vi "InstrumentControlExercises_MichaelVasmerDavidWise.vi"() -> ()   [LabVIEW 2012]
doc: "This example shows how to configure a measurement and take a reading."
uses:
  Program Files (x86)/National Instruments/LabVIEW 2013/instr.lib/Keithley 24XX/Keithley 24XX.lvlib
  <vilib>/express/express arith-compare/Formula/XNode/ExpressFormulaBlockNode.xnode
  Control2_MichaelVasmerDavidWise.ctl
  He3_Tlogger_Global 1.vi
  Control3_MichaelVasmerDavidWise.ctl
  Program Files (x86)/National Instruments/LabVIEW 2013/instr.lib/Stanford Research 830/Stanford Research 830.lvlib
  Program Files (x86)/National Instruments/LabVIEW 2013/instr.lib/Keithley 24XX/Public/Data/Read (Single Point).vi
  Program Files (x86)/National Instruments/LabVIEW 2013/instr.lib/Stanford Research 830/Public/Data/Read (All Parameters).vi
  <vilib>/Utility/file.llb/Write To Spreadsheet File (string).vi
  <vilib>/Utility/file.llb/Write To Spreadsheet File (DBL).vi
panel:
  out "Step constant":dbl
  out "Forwards":bool
  out "Array":dbl[](array[numeric])=[0.002, 0.004, 0.006, 0.008, 0.01, 0.012, 0.014, 0.016, 0.018000000000000002, 0.02, 0.022, 0.024, 0.026000000000000002, 0.028]
  out "error out":errorcluster
  out "VISA resource name out":refnum<visa-resource-name>="Keithley"
  in  "Compliance  Level (0.1)":dbl=4.0
  out "Keithley Input Current (A)":dbl=0.4222222222222222
  out "T 2":dbl=293.425
  out "T 1":dbl=293.425
  out "V_output_Y_channel":dbl
  out "V_output_X_channel":dbl=0.0153199
  in  "R Series Value":dbl=100000.0
  in  "True  = R(B)\nFalse = R(T)":bool
  in  "Lock In On (default false)":bool
  out "Outer State Machine":T1=enum."Idle"
  out "Inner State Machine":T2=enum."Idle"
  out "I_AC Amplitude (A)":dbl=1e-05
  in  "Keithley on (default false)":bool
  out "Magnetic Field (T)":dbl
  in  "Internal Reference Frequency (1000 Hz)":dbl=1573.0
  in  "Sine Output Amplitude (1 V)":dbl=1.0
  in  "Sensitivity (26: 1 V/uA)":i8(ring)=26 items=["Auto Gain"=-1, "2 nV/fA"=0, "5 nV/fA"=1, "10 nV/fA"=2, "20 nV/fA"=3, "50 nV/fA"=4, "100 nV/fA"=5, "200 nV/fA"=6, "500 nV/fA"=7, "1 uV/pA"=8, "2 uV/pA"=9, "5 uV/pA"=10, "10 uV/pA"=11, "20 uV/pA"=12, "50 uV/pA"=13, "100 uV/pA"=14, "200 uV/pA"=15, "500 uV/pA"=16, "1 mV/nA"=17, "2 mV/nA"=18, "5 mV/nA"=19, "10 mV/nA"=20, "20 mV/nA"=21, "50 mV/nA"=22, "100 mV/nA"=23, "200 mV/nA"=24, "500 mV/mA"=25, "1 V/uA"=26]
  in  "Dynamic Reserve (2: Low Noise)":i8(ring)=2 items=["High Reserve"=0, "Normal"=1, "Low Noise"=2, "Auto Reserve"=-1]
  in  "Reference Source (1: Internal)":u16(ring)=1 items=["External", "Internal"]
  in  "Input Coupling (0: AC)":u16(ring) items=["AC", "DC"]
  in  "Input Connection (0: Single-Ended Voltage)":u16(ring) items=["Single-Ended Voltage", "Differential Voltage", "1 MOhm Current Gain", "100 MOhm Current Gain"]
  in  "VISA resource name Lock-In":refnum<visa-resource-name>="LockIn"
  out "Temperature (K)":dbl=293.453
  in  "Shutdown":bool
  out "Resistance":sgl=13619.99
  out "Current":sgl=0.00029368006
  out "Voltage":sgl=3.9999197
  in  "Enable Resistance Auto Range (T:Enable)":bool=TRUE
  in  "Enable Current Auto Range (T:Enable)":bool=TRUE
  in  "Enable Voltage Auto Range (T:Enable)":bool=TRUE
  in  "Resistance Manual Range (1.0)":dbl=1.0
  in  "Current Manual Range (1.0)":dbl=1.0
  in  "Voltage Manual Range (1.0)":dbl=1.0
  in  "Serial Configuration":T3={"Baud Rate"=9600, "Parity"=0, "Data Bits"=8, "Stop Bits"=10, "Flow Control"=0} {"Flow Control" items=["None", "XON/XOFF", "RTS/CTS", "XON/XOFF & RTS/CTS", "DTR/DSR", "XON/XOFF & DTR/DSR"]; "Stop Bits" items=["1.0"=10, "1.5"=15, "2.0"=20]; "Data Bits" items=["7"=7, "8"=8]; "Parity" items=["None", "Odd", "Even", "Mark", "Space"]; "Baud Rate" items=["300"=300, "600"=600, "1200"=1200, "2400"=2400, "4800"=4800, "9600"=9600, "19200"=19200]}
  in  "VISA resource name Kiethley":refnum<visa-resource-name>="Keithley"
  in  "Tab Control":enum32{" R(B)", "R(T)"}(tab)=enum."R(T)"
  in  "Time Delay":dbl=2.0
  out "Field too high error":string
  in  "Sweep R(B)":bool
  in  "B Max\n|B|<0.0716":dbl=0.03 step=0.01
  in  "File String Template":string="C:\\Users\\Josephson Lab User\\Documents\\CDT_2016\\MichaelDavid\\data\\test_RB"
  out "R vs B":cluster{dbl[], dbl[]}(graph)={[0.002, 0.004, 0.006, 0.008, 0.01, 0.012, 0.014, 0.016, 0.018000000000000002, 0.02, 0.022, 0.024, 0.026000000000000002, 0.028, 0.029999999999999995], [1531.9899999999998, 1531.9899999999998, 1531.9899999999998, 1531.9899999999998, 1531.9899999999998, 1531.9899999999998, 1531.9899999999998, 1531.9899999999998, 1531.9899999999998, 1531.9899999999998, 1531.9899999999998, 1531.9899999999998, 1531.9899999999998, 1531.9899999999998, 1531.9899999999998]}
  in  "Steps":dbl=15.0
  in  "Sweep R(T)":bool
  in  "Stop Sweep R(T)":bool
  in  "Force Measurement":bool
  in  "File String Template 2":string="C:\\Users\\Josephson Lab User\\Documents\\CDT_2016\\MichaelDavid\\data\\test_RT"
  out "R vs Temp":cluster{dbl[], dbl[]}(graph)={[293.427, 293.452, 293.456, 293.434, 293.429, 293.426, 293.438, 293.446, 293.454, 293.431, 293.461, 293.42, 293.423, 293.447, 293.466, 293.452, 293.463, 293.456, 293.44, 293.45, 293.434, 293.442, 293.425], [1531.9899999999998, 1531.9899999999998, 1531.9899999999998, 1531.9899999999998, 1531.9899999999998, 1531.9899999999998, 1531.9899999999998, 1531.9899999999998, 1531.9899999999998, 1531.9899999999998, 1531.9899999999998, 1531.9899999999998, 1531.9899999999998, 1531.9899999999998, 1531.9899999999998, 1531.9899999999998, 1531.9899999999998, 1531.9899999999998, 1531.9899999999998, 1531.9899999999998, 1531.9899999999998, 1531.9899999999998, 1531.9899999999998]}
  # "Keithley Settings"
  # "Voltage Range Settings"
  # "Current Range Settings"
  # "Resistance Range Settings"
  # "SR830 Lock In Settings"
  # "Keithley Output"
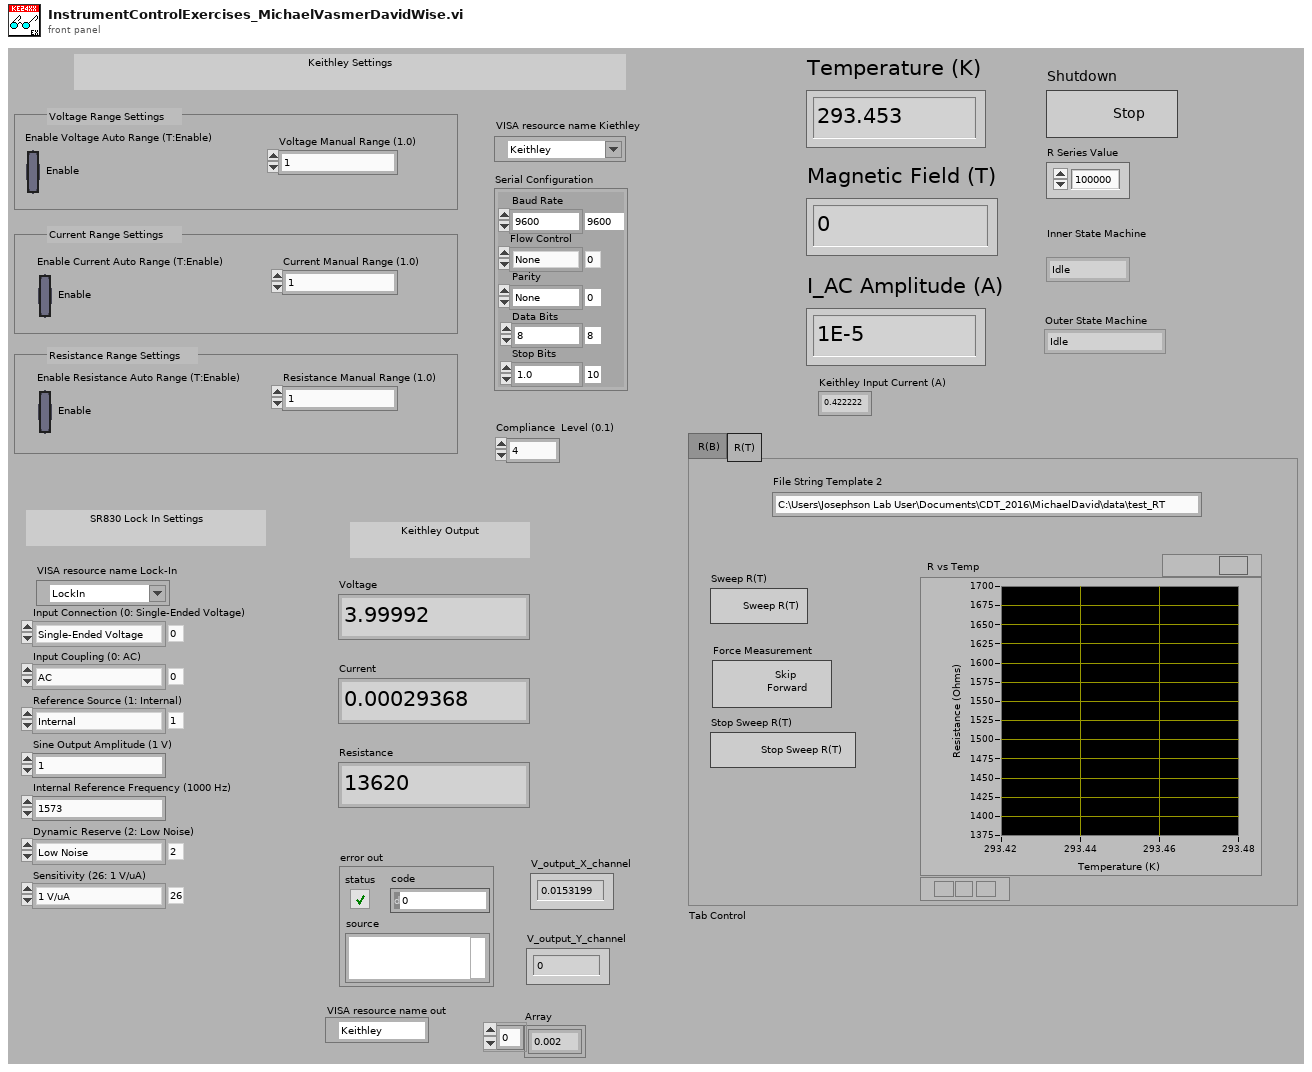
[diagram p1: front panel]
types:
  T1 = typedef "Control2_MichaelVasmerDavidWise.ctl" = enum16{"Open File 2", "Write File", "Open File", "Shutdown All", "Shutdown Lock in", "Read R(T)", "Init Lock In", "Increment", "Shutdown Keithley", "Idle", "Exit", "Read R(B)", "Set B", "Init Keithley"}
  T2 = typedef "Control3_MichaelVasmerDavidWise.ctl" = enum16{"Write File", "Read T 2", "Idle", "Read Lockin", "Read T"}
  T3 = cluster{"Baud Rate":u32, "Parity":u16, "Data Bits":u16, "Stop Bits":u16, "Flow Control":u16}
  T4 = cluster{"X-Value":dbl, "Y-Value":dbl, "R-Value":dbl, "Theta-Value":dbl, "Aux In 1 Value":dbl, "Aux In 2 Value":dbl, "Aux In 3 Value":dbl, "Aux In 4 Value":dbl, "Reference Frequency":dbl, "Channel 1 Display":dbl, "Channel 2 Display":dbl}
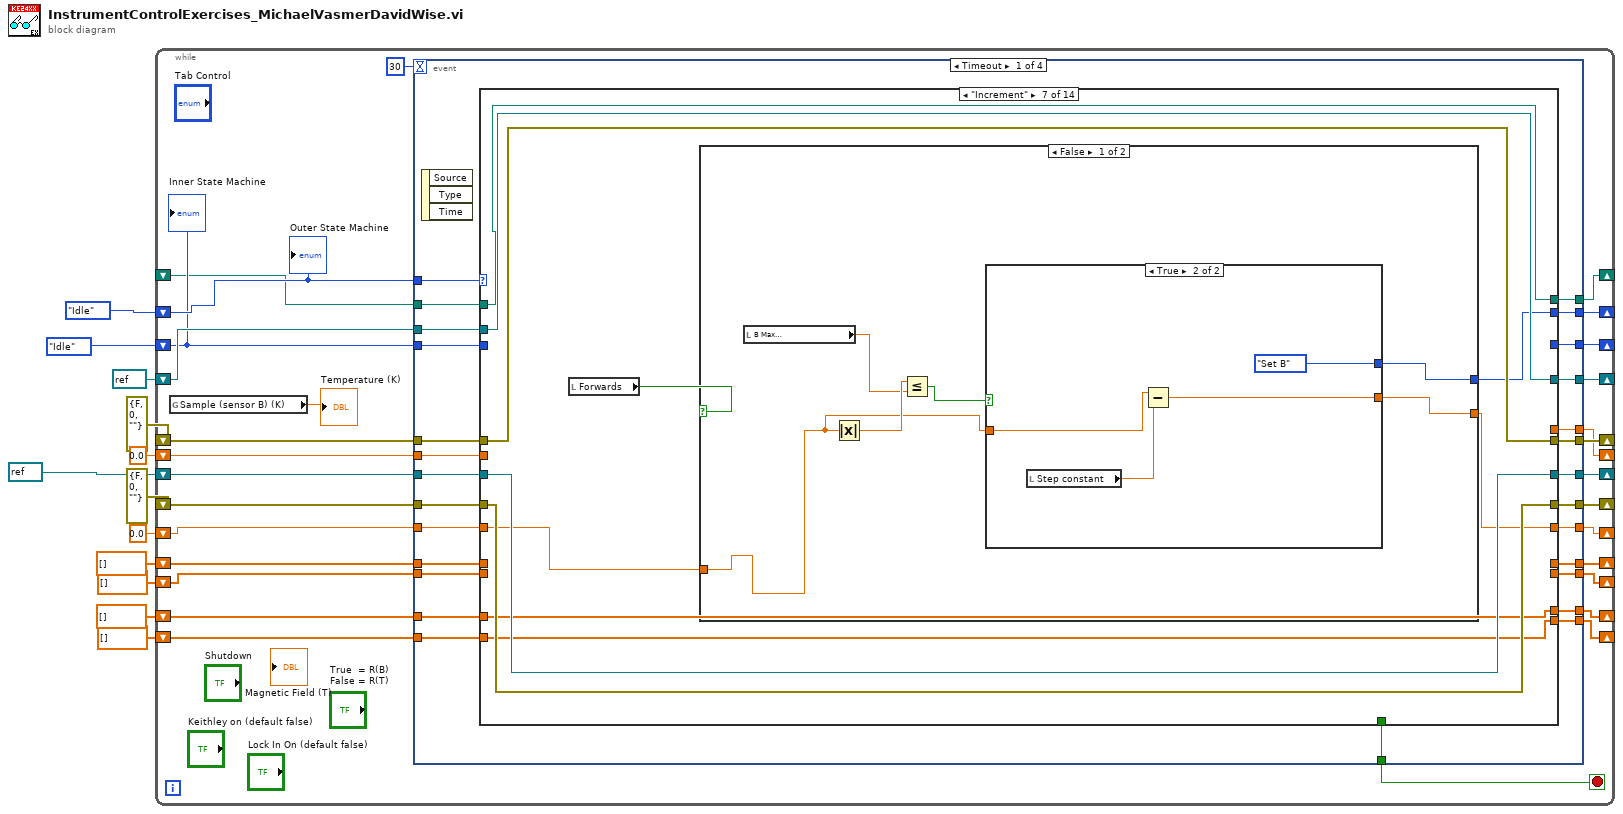
[diagram p0: block diagram]
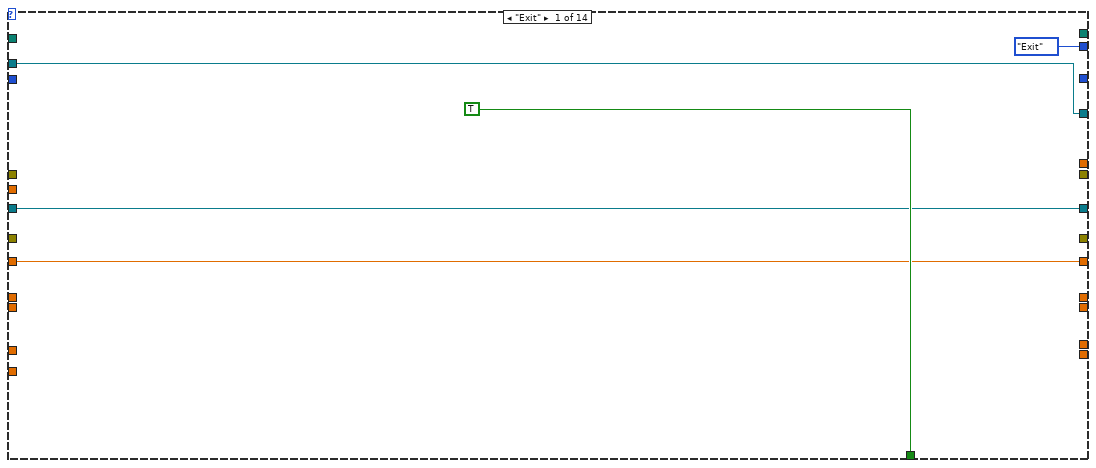
[diagram p2: hidden frame]
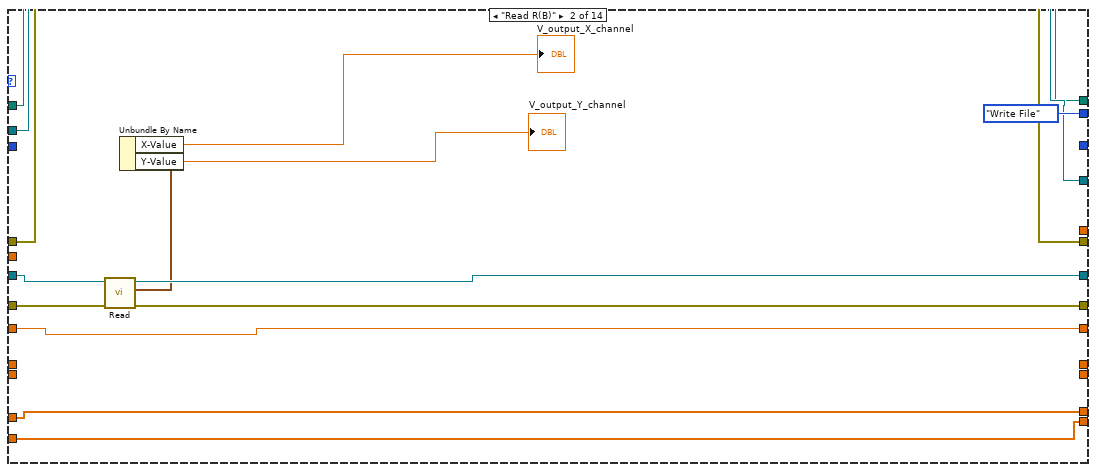
[diagram p3: hidden frame]
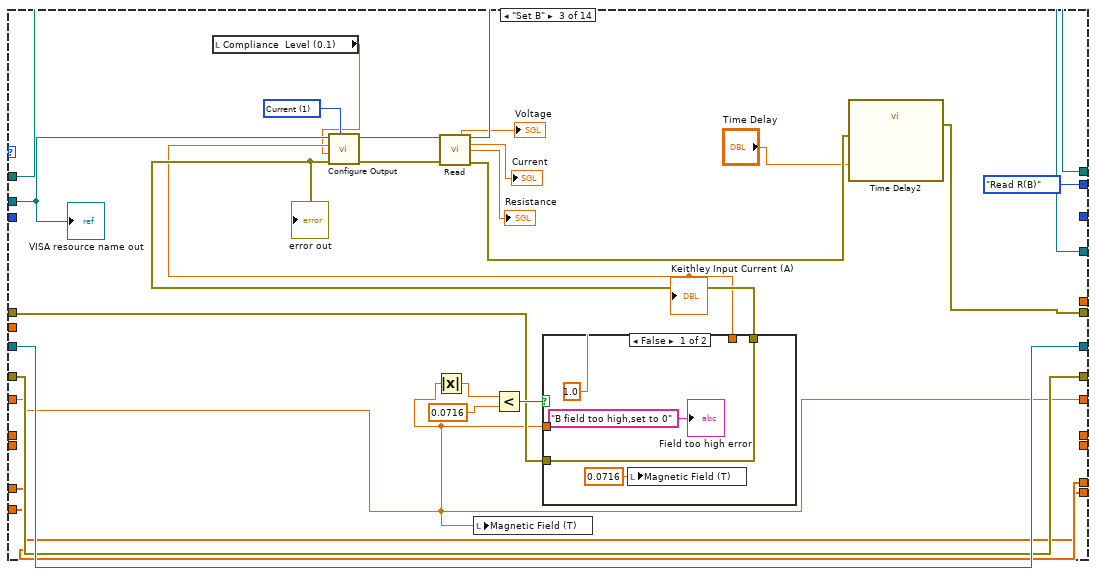
[diagram p4: hidden frame]
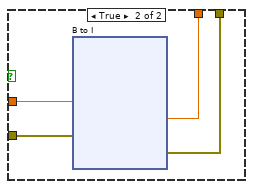
[diagram p5: hidden frame]
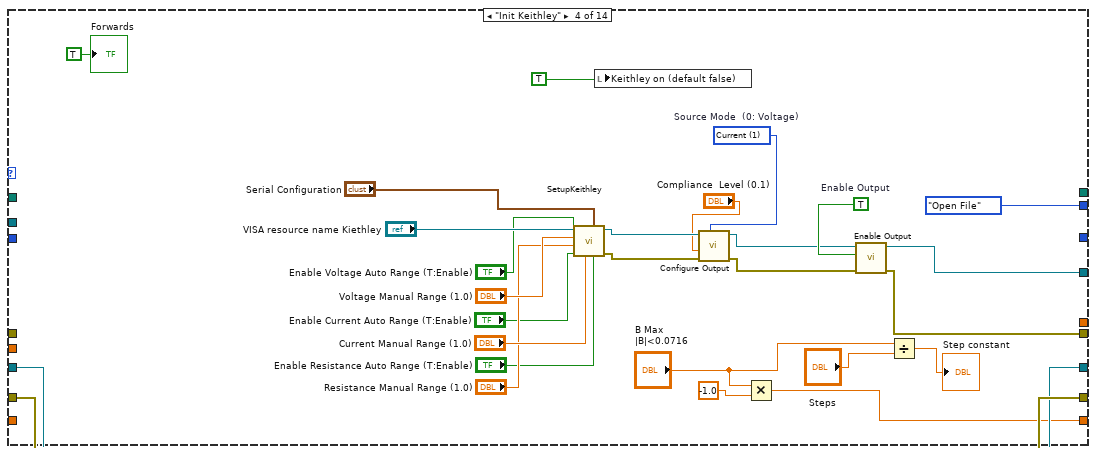
[diagram p6: hidden frame]
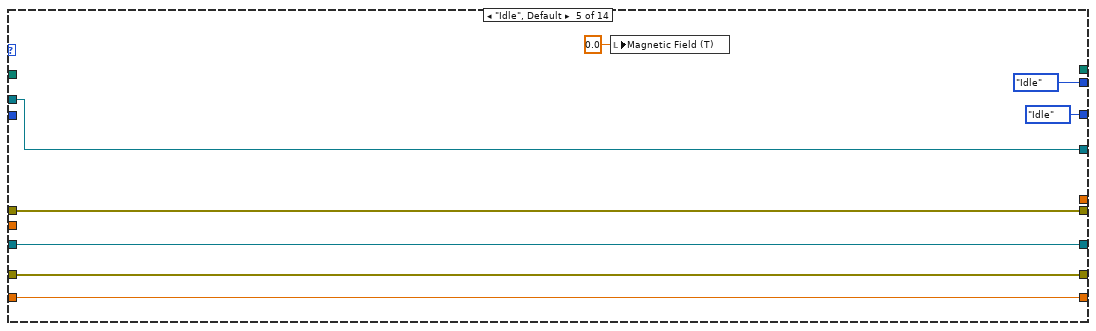
[diagram p7: hidden frame]
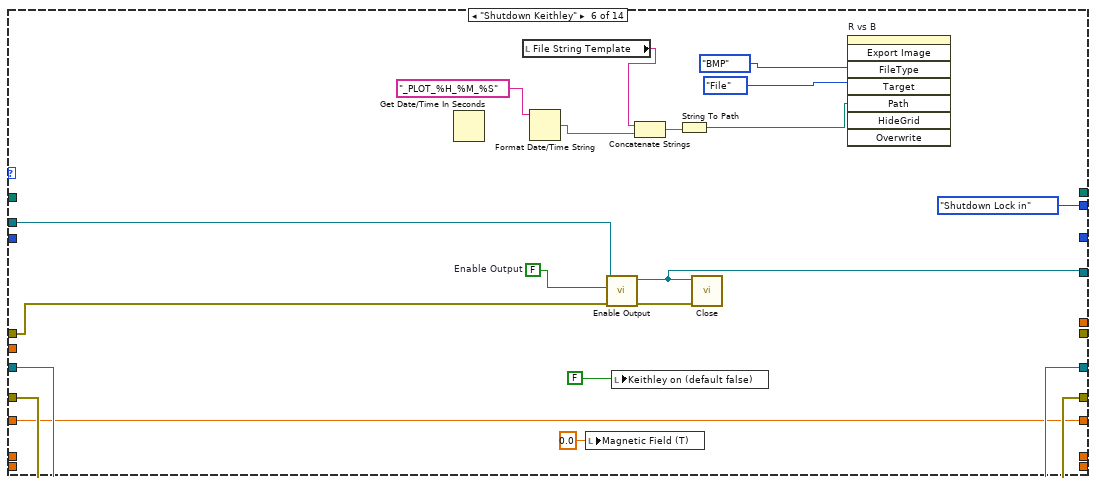
[diagram p8: hidden frame]
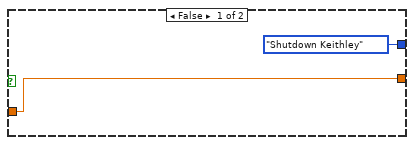
[diagram p9: hidden frame]
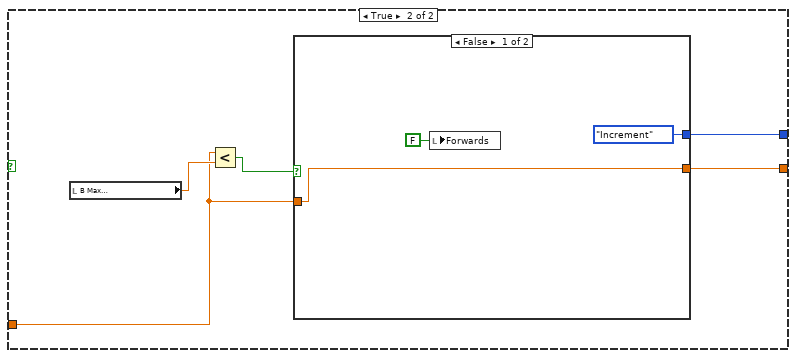
[diagram p10: hidden frame]
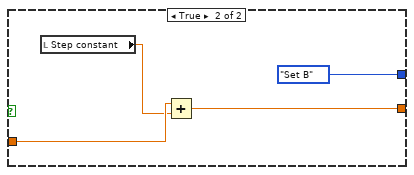
[diagram p11: hidden frame]
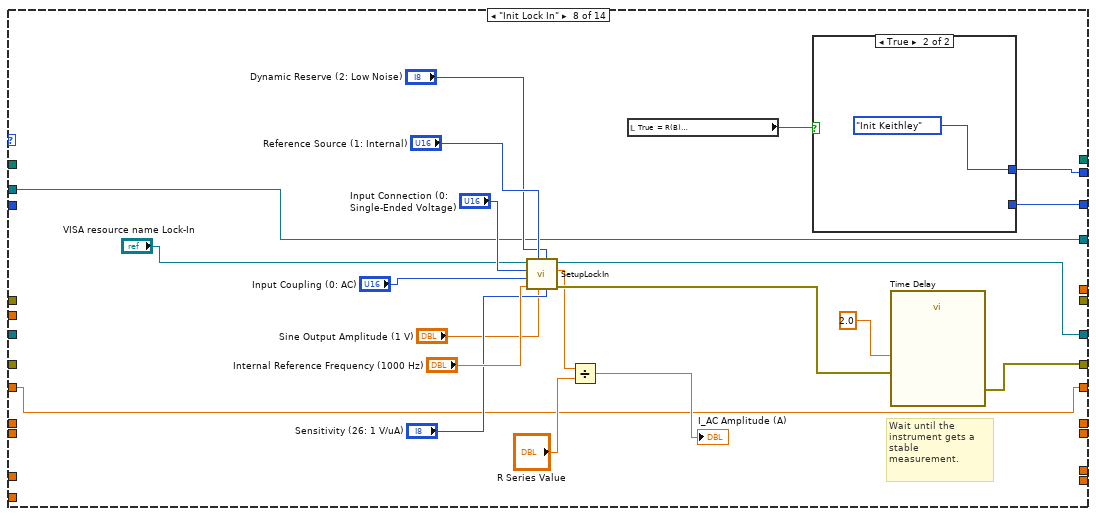
[diagram p12: hidden frame]
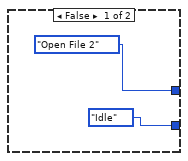
[diagram p13: hidden frame]
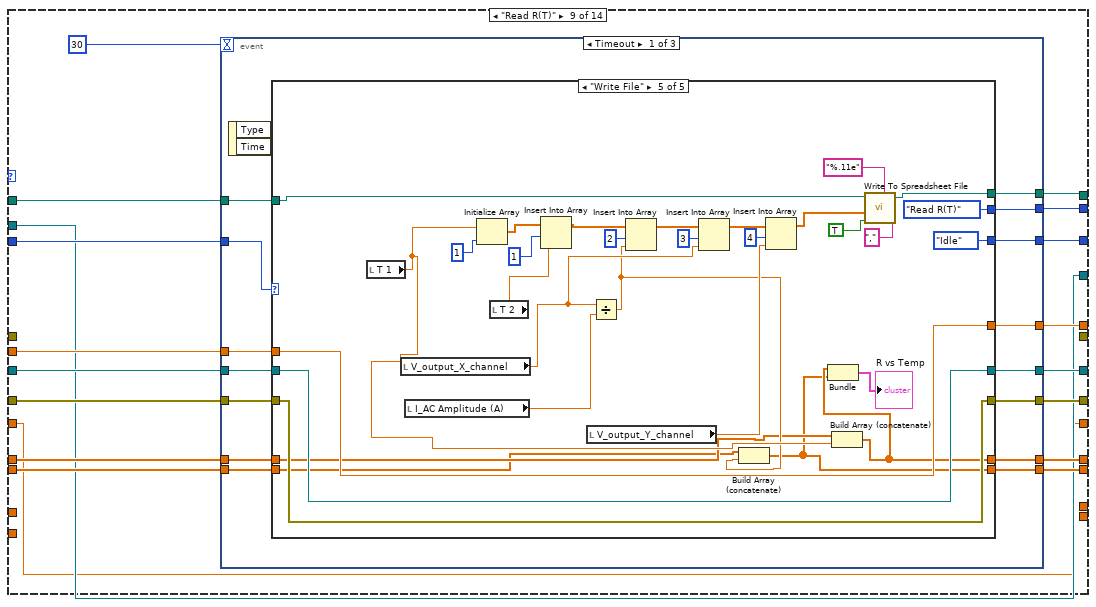
[diagram p14: hidden frame]
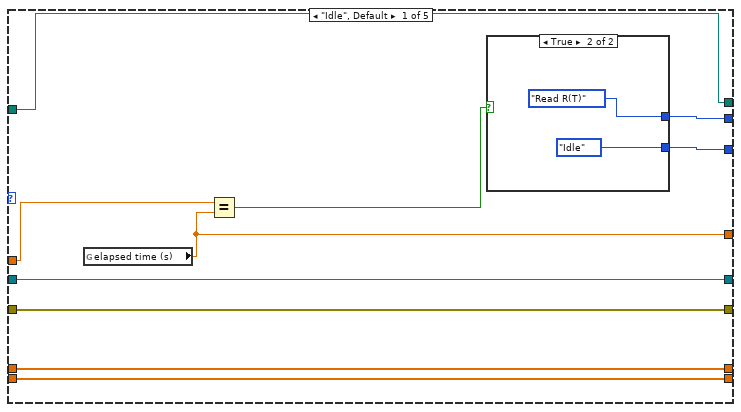
[diagram p15: hidden frame]
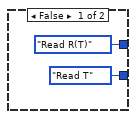
[diagram p16: hidden frame]
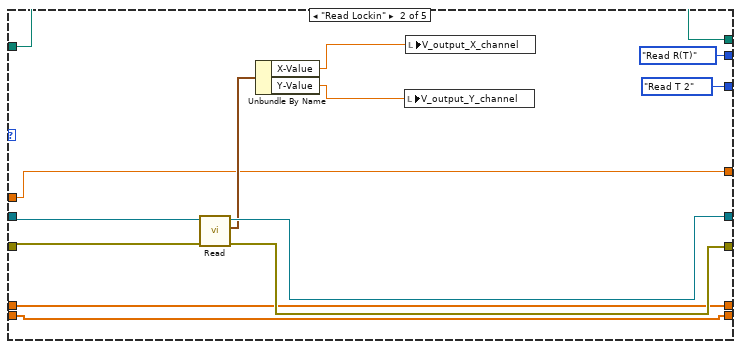
[diagram p17: hidden frame]
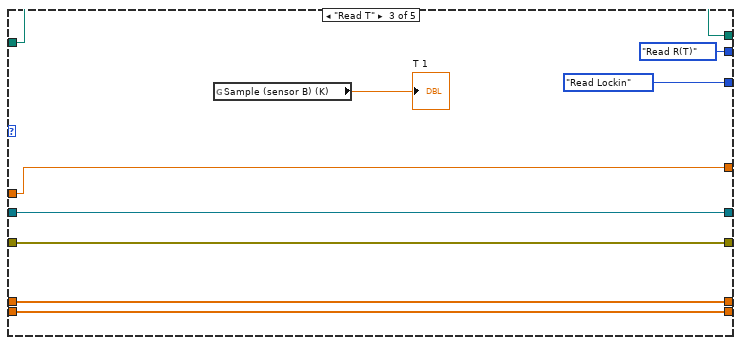
[diagram p18: hidden frame]
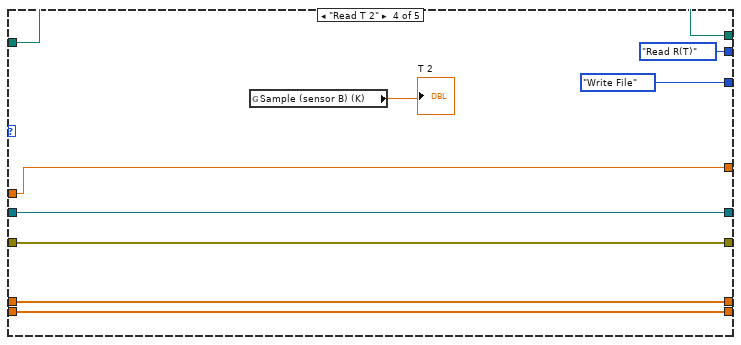
[diagram p19: hidden frame]
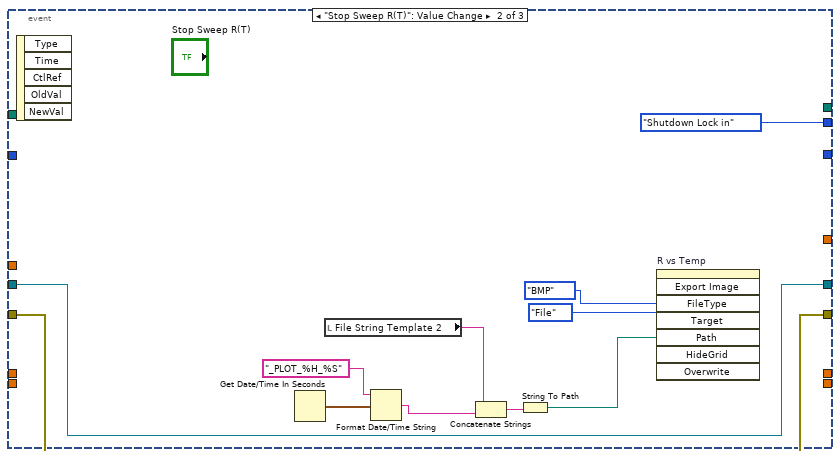
[diagram p20: hidden frame]
diagram:
  n1 = while {
    shift-right: [w40] -> _
    shift-left: Control2_MichaelVasmerDavidWise."Idle" -> [w41]
    shift-right: [w39] -> _
    shift-left: refnum<visa-resource-name> refnum ("VISA resource name out") -> [w36]
    shift-right: [w38] -> _
    shift-left: errorcluster {"status"=FALSE, "code"=0, "source"=""} ("error out") -> [w35]
    shift-right: [w33] -> _
    shift-left: Control3_MichaelVasmerDavidWise."Idle" -> [w27]
    shift-right: [w32] -> _
    shift-left: refnum<visa-resource-name> refnum ("VISA resource name out") -> [w29]
    shift-right: [w31] -> _
    shift-left: errorcluster {"status"=FALSE, "code"=0, "source"=""} ("error out") -> [w30]
    shift-right: [w26] -> _
    shift-left: _ -> [w25]
    shift-right: [w23] -> _
    shift-left: 0.0 ("elapsed time (s)") -> [w24]
    shift-right: [w22] -> _
    shift-left: dbl[] [] -> [w20]
    shift-right: [w21] -> _
    shift-left: dbl[] [] -> [w19]
    shift-right: [w16] -> _
    shift-left: dbl[] [] -> [w18]
    shift-right: [w15] -> _
    shift-left: dbl[] [] -> [w17]
    shift-right: [w14] -> _
    shift-left: 0.0 -> [w13]
    stop <- w34 stop-if-true
    n2 = global read "He3_Tlogger_Global 1.vi" "Sample (sensor B) (K)"() -> (→"Temperature (K)":dbl)
    n3 = event shown="[0] Timeout" {
      selector: _ -> [_ _ _ _]
      dyn-events: _ -> [_ _ _ _]
      timeout: 30 -> [_ _ _ _]
      tunnel: w41 -> [w68 _ _ _]
      tunnel: [w67 Control2_MichaelVasmerDavidWise."Shutdown All" Control2_MichaelVasmerDavidWise."Init Lock In" Control2_MichaelVasmerDavidWise."Init Lock In"] -> w40
      tunnel: [w66 w514 w517 w522] -> w39
      tunnel: [w65 _ _ _] -> w38
      tunnel: w36 -> [w64 w514 w517 w522]
      tunnel: w35 -> [w63 _ _ _]
      tunnel: [w62 _ _ _] -> w34
      tunnel: w27 -> [w61 _ _ _]
      tunnel: [w60 _ Control3_MichaelVasmerDavidWise."Idle" _] -> w33
      tunnel: [w59 w513 w516 w521] -> w32
      tunnel: [w58 _ _ _] -> w31
      tunnel: w30 -> [w57 _ _ _]
      tunnel: w29 -> [w56 w513 w516 w521]
      tunnel: [w55 _ _ _] -> w26
      tunnel: w25 -> [w54 _ _ _]
      tunnel: w24 -> [w53 _ _ _]
      tunnel: [w52 _ _ _] -> w23
      tunnel: [w51 _ _ _] -> w22
      tunnel: [w50 _ _ _] -> w21
      tunnel: w20 -> [w49 _ _ _]
      tunnel: w19 -> [w48 _ _ _]
      tunnel: w18 -> [w47 _ _ _]
      tunnel: w17 -> [w46 _ _ _]
      tunnel: [w45 _ _ _] -> w16
      tunnel: [w44 _ _ _] -> w15
      tunnel: [w43 _ _ _] -> w14
      tunnel: w13 -> [w42 _ _ _]
      event Timeout {
        n4 = event-data() -> ()  [unwired: 1 in, 3 out]
        n5 = case shown="\"Increment\"" w68 {
          tunnel: [Control2_MichaelVasmerDavidWise."Exit" Control2_MichaelVasmerDavidWise."Write File" Control2_MichaelVasmerDavidWise."Read R(B)" Control2_MichaelVasmerDavidWise."Open File" Control2_MichaelVasmerDavidWise."Idle" Control2_MichaelVasmerDavidWise."Shutdown Lock in" w182 w229 w254 Control2_MichaelVasmerDavidWise."Exit" Control2_MichaelVasmerDavidWise."Idle" Control2_MichaelVasmerDavidWise."Set B" Control2_MichaelVasmerDavidWise."Increment" Control2_MichaelVasmerDavidWise."Read R(T)"] -> w67
          tunnel: [w71 w82 w100 w147 w162 w168 w192 w218 w241 w370 w391 w397 w464 w470] -> w66
          tunnel: [_ w81 w90 w144 w163 _ w191 _ _ _ _ _ w465 _] -> w65
          tunnel: w64 -> [w71 w82 w96 _ w162 w176 w192 w218 w241 w374 w391 w397 w464 w470]
          tunnel: w63 -> [_ w81 w101 _ w163 w180 w191 _ _ w375 _ _ w465 _]
          tunnel: [TRUE _ _ _ _ _ _ _ _ _ _ _ _ _] -> w62
          tunnel: w61 -> [_ _ _ _ _ _ _ _ w256 _ _ _ _ _]
          tunnel: [_ _ _ _ Control3_MichaelVasmerDavidWise."Idle" _ _ w219 w255 _ _ _ _ Control3_MichaelVasmerDavidWise."Idle"] -> w60
          tunnel: [w70 w86 w106 w142 w159 w173 w189 w228 w250 w369 w390 w396 w466 w473] -> w59
          tunnel: [_ w85 w105 w143 w158 w174 w190 w226 w251 _ _ _ w467 w474] -> w58
          tunnel: w57 -> [_ w84 w105 w143 w158 w174 w190 _ w253 w372 w394 _ w467 w474]
          tunnel: w56 -> [w70 w80 w106 w142 w159 w173 w189 _ w252 w373 w390 w396 w466 w473]
          tunnel: [_ w79 w97 _ _ _ w188 _ w249 _ _ w409 w446 w472] -> w55
          tunnel: w54 -> [_ w79 w97 _ _ _ w188 _ w248 _ _ _ w461 _]
          tunnel: w53 -> [_ _ _ _ _ _ _ _ w247 _ _ _ _ _]
          tunnel: [_ _ _ _ _ _ _ _ w246 _ _ _ _ _] -> w52
          tunnel: [_ _ _ _ _ _ _ _ w245 _ _ _ _ _] -> w51
          tunnel: [_ _ _ _ _ _ _ _ w244 _ _ _ _ _] -> w50
          tunnel: w49 -> [_ _ _ _ _ _ _ _ w243 _ _ _ _ _]
          tunnel: w48 -> [_ _ _ _ _ _ _ _ w242 _ _ _ _ _]
          tunnel: w47 -> [_ w76 w93 _ _ _ w187 _ _ _ _ _ w444 _]
          tunnel: w46 -> [_ w75 w92 _ _ _ w186 _ _ _ _ _ w443 _]
          tunnel: [_ w76 w93 _ _ _ w187 _ _ _ _ _ w440 _] -> w45
          tunnel: [_ w75 w92 _ _ _ w186 _ _ _ _ _ w439 _] -> w44
          tunnel: [w69 w74 w88 w129 w156 w164 w183 w217 w240 w368 w389 w395 w437 w469] -> w43
          tunnel: w42 -> [w69 w74 w88 _ w156 w164 w184 w217 w240 w368 w389 w395 w437 w469]
          frame "Exit" {
          }
          frame "Read R(B)" {
            n6 = call-poly "Read.vi"("error in (no error)"=w84, "VISA resource name"=w80) -> ("error out"=w85:errorcluster, "Parameter Values"=w83:T4, "VISA resource name out"=w86:refnum<visa-resource-name>)  [unwired: 7 in]
            n7 = Unbundle By Name(w83) -> ("X-Value"=→"V_output_X_channel":dbl, "Y-Value"=→"V_output_Y_channel":dbl)
          }
          frame "Set B" {
            w95 = u16 1 items=["Voltage", "Current"] ("Source Mode  (0: Voltage)")
            n8 = local read "Compliance  Level (0.1)"() -> (w94:dbl)
            n9 = Absolute Value(x=w88) -> (abs(x)=w98:dbl)
            n10 = local write "Magnetic Field (T)"(w88) -> ()
            n11 = Less?(x=w98, y=0.0716 ("x")) -> (x < y?=w108:bool)
            n12 = case shown="False" w108 {
              tunnel: w88 -> [_ w120]
              tunnel: [1.0 ("x") w119] -> w102
              tunnel: w101 -> [w115 w118]
              tunnel: [w115 w117] -> w104
              frame False {
                n13 = local write "Magnetic Field (T)"(0.0716 ("Magnetic Field (T)")) -> ()
                "Field too high error" <- "B field too high,set to 0" ("String")
              }
              frame True {
                n14 = xnode "B to I"("X1"=w120, "error in (no error)"=w118) -> ("Result"=w119:dbl, "error out"=w117:errorcluster)
              }
            }
            "Keithley Input Current (A)" <- w102
            "error out" <- w104
            n15 = call "Configure Output.vi"("Source Mode  (0: Voltage)"=w95, "error in (no error)"=w104, "Compliance  Level (0.1)"=w94, "Output Level (0)"=w102, "VISA resource name"=w96) -> ("error out"=w109:errorcluster, "VISA resource name out"=w110:refnum<visa-resource-name>)  [unwired: 5 in]
            n16 = call-poly "Read.vi"("VISA resource name"=w110, "error in (no error)"=w109) -> ("Voltage"=→"Voltage":sgl, "VISA resource name out"=w100:refnum<visa-resource-name>, "Current"=→"Current":sgl, "Resistance"=→"Resistance":sgl, "error out"=w91:errorcluster)  [unwired: 7 in, 2 out]
            n17 = call "Time Delay2"("error in (no error)"=w91, "Delay Time (s)"="Time Delay") -> ("error out"=w90:errorcluster)  [unwired: 9 in]
            "VISA resource name out" <- w96
          }
          frame "Init Keithley" {
            w135 = u16 1 items=["Voltage", "Current"]  # Source Mode  (0: Voltage)
            w148 = TRUE  # Enable Output
            n18 = call "SetupKeithley.vi"("Enable Resistance Auto Range (T:Enable)"="Enable Resistance Auto Range (T:Enable)", "Serial Configuration"="Serial Configuration", "Current Manual Range (1.0)"="Current Manual Range (1.0)", "Enable Voltage Auto Range (T:Enable)"="Enable Voltage Auto Range (T:Enable)", "Enable Current Auto Range (T:Enable)"="Enable Current Auto Range (T:Enable)", "Resistance Manual Range (1.0)"="Resistance Manual Range (1.0)", "Voltage Manual Range (1.0)"="Voltage Manual Range (1.0)", "VISA Refnum in"="VISA resource name Kiethley") -> ("error out"=w137:errorcluster, "VISA Refnum out"=w138:refnum<visa-resource-name>)  [unwired: 2 in]
            n19 = local write "Keithley on (default false)"(TRUE ("Keithley on")) -> ()
            n20 = call "Configure Output.vi"("Source Mode  (0: Voltage)"=w135, "error in (no error)"=w137, "Compliance  Level (0.1)"="Compliance  Level (0.1)", "VISA resource name"=w138) -> ("error out"=w139:errorcluster, "VISA resource name out"=w140:refnum<visa-resource-name>)  [unwired: 6 in]
            n21 = Multiply(x="B Max\n|B|<0.0716", y=-1.0) -> (x*y=w129:dbl)
            n22 = call "Enable Output.vi"("error in (no error)"=w139, "Enable Output (T: Enable)"=w148, "VISA resource name"=w140) -> ("error out"=w144:errorcluster, "VISA resource name out"=w147:refnum<visa-resource-name>)  [unwired: 7 in]
            n23 = Divide(x="B Max\n|B|<0.0716", y="Steps") -> (x/y=→"Step constant":dbl)
            "Forwards" <- TRUE ("Forwards")
          }
          frame "Idle", Default {
            n24 = local write "Magnetic Field (T)"(0.0 ("Magnetic Field (T)")) -> ()
          }
          frame "Shutdown Keithley" {
            w175 = FALSE  # Enable Output
            n25 = Get Date/Time In Seconds() -> ()  [unwired: 1 out]
            n26 = local read "File String Template"() -> (w170:string)
            n27 = Format Date/Time String(time format string (%c)="_PLOT_%H_%M_%S") -> (date/time string=w169:string)  [unwired: 2 in]
            n28 = local write "Magnetic Field (T)"(0.0 ("Magnetic Field (T)")) -> ()
            n29 = call "Enable Output.vi"("error in (no error)"=w180, "Enable Output (T: Enable)"=w175, "VISA resource name"=w176) -> ("error out"=w181:errorcluster, "VISA resource name out"=w168:refnum<visa-resource-name>)  [unwired: 7 in]
            n30 = local write "Keithley on (default false)"(FALSE ("Keithley on")) -> ()
            n31 = Concatenate Strings(w170, w169) -> (w172:string)
            n32 = String To Path(string=w172) -> (path=w165:path)
            n33 = call "Close.vi"("error in (no error)"=w181, "VISA resource name"=w168) -> ()  [unwired: 9 in, 1 out]
            n34 = invoke on="R vs B" class="XYGraph (strict)" method="Export Image"("FileType"=enum32{"BMP", "EPS", "EMF", "PICT"}."BMP" ("File Type"), "Target"=enum32{"File", "Clipboard"}."File", "Path"=w165) -> ()  [unwired: 5 in, 8 out]
          }
          frame "Increment" {
            n35 = local read "Forwards"() -> (w185:bool)
            n36 = case shown="False" w185 {
              tunnel: w184 -> [w194 w207]
              tunnel: [w196 w206] -> w183
              tunnel: [w197 w205] -> w182
              frame False {
                n37 = local read "B Max\n|B|<0.0716"() -> (w193:dbl)
                n38 = Absolute Value(x=w194) -> (abs(x)=w195:dbl)
                n39 = Less Or Equal?(x=w195, y=w193) -> (x <= y?=w198:bool)
                n40 = case shown="True" w198 {
                  tunnel: w194 -> [w200 w204]
                  tunnel: [w200 w203] -> w196
                  tunnel: [Control2_MichaelVasmerDavidWise."Shutdown Keithley" Control2_MichaelVasmerDavidWise."Set B"] -> w197
                  frame False {
                  }
                  frame True {
                    n41 = local read "Step constant"() -> (w201:dbl)
                    n42 = Subtract(x=w204, y=w201) -> (x-y=w203:dbl)
                  }
                }
              }
              frame True {
                n43 = local read "B Max\n|B|<0.0716"() -> (w209:dbl)
                n44 = Less?(x=w207, y=w209) -> (x < y?=w208:bool)
                n45 = case shown="False" w208 {
                  tunnel: w207 -> [w211 w216]
                  tunnel: [w211 w214] -> w206
                  tunnel: [Control2_MichaelVasmerDavidWise."Increment" Control2_MichaelVasmerDavidWise."Set B"] -> w205
                  frame False {
                    n46 = local write "Forwards"(FALSE ("Forwards")) -> ()
                  }
                  frame True {
                    n47 = local read "Step constant"() -> (w215:dbl)
                    n48 = Add(x=w216, y=w215) -> (x+y=w214:dbl)
                  }
                }
              }
            }
          }
          frame "Init Lock In" {
            # "Wait until the instrument gets a stable measurement."
            n49 = call "SetupLockIn.vi"("Sensitivity (26: 1 V/uA)"="Sensitivity (26: 1 V/uA)", "Dynamic Reserve (2: Low Noise)"="Dynamic Reserve (2: Low Noise)", "Sine Output Amplitude (1 V)"="Sine Output Amplitude (1 V)", "Reference Source (1: Internal)"="Reference Source (1: Internal)", "Internal Reference Frequency (1000 Hz)"="Internal Reference Frequency (1000 Hz)", "Input Coupling (0: AC)"="Input Coupling (0: AC)", "Input Connection (0: Single-Ended Voltage)"="Input Connection (0: Single-Ended Voltage)", "VISA Refnum in"="VISA resource name Lock-In") -> ("error out"=w227:errorcluster, "V_AC Amplitude (A)"=w222:dbl, "VISA Refnum out"=w228:refnum<visa-resource-name>)  [unwired: 1 in]
            n50 = Divide(x=w222, y="R Series Value") -> (x/y=→"I_AC Amplitude (A)":dbl)
            n51 = local read "True  = R(B)\nFalse = R(T)"() -> (w223:bool)
            n52 = case shown="True" w223 {
              tunnel: [Control2_MichaelVasmerDavidWise."Open File 2" Control2_MichaelVasmerDavidWise."Init Keithley"] -> w229
              tunnel: [Control3_MichaelVasmerDavidWise."Idle" _] -> w219
              frame False {
              }
              frame True {
              }
            }
            n53 = call "Time Delay"("error in (no error)"=w227, "Delay Time (s)"=2.0) -> ("error out"=w226:errorcluster)  [unwired: 9 in]
          }
          frame "Read R(T)" {
            n54 = event shown="[0] Timeout" {
              selector: _ -> [_ _ _]
              dyn-events: _ -> [_ _ _]
              timeout: 30 -> [_ _ _]
              tunnel: w256 -> [w272 _ _]
              tunnel: [w271 _ Control3_MichaelVasmerDavidWise."Read T"] -> w255
              tunnel: [w264 Control2_MichaelVasmerDavidWise."Shutdown Lock in" Control2_MichaelVasmerDavidWise."Read R(T)"] -> w254
              tunnel: w253 -> [w270 w353 w363]
              tunnel: w252 -> [w269 w352 w364]
              tunnel: [w268 w353 w363] -> w251
              tunnel: [w267 w352 w364] -> w250
              tunnel: [w266 _ w365] -> w249
              tunnel: w248 -> [w265 _ w365]
              tunnel: w247 -> [w263 _ w362]
              tunnel: [w262 _ w362] -> w246
              tunnel: [w261 _ w361] -> w245
              tunnel: [w260 _ w360] -> w244
              tunnel: w243 -> [w259 _ w361]
              tunnel: w242 -> [w258 _ w360]
              event Timeout {
                n55 = event-data() -> ()  [unwired: 1 in, 2 out]
                n56 = case shown="\"Write File\"" w272 {
                  tunnel: [w282 Control3_MichaelVasmerDavidWise."Read T 2" Control3_MichaelVasmerDavidWise."Read Lockin" Control3_MichaelVasmerDavidWise."Write File" Control3_MichaelVasmerDavidWise."Idle"] -> w271
                  tunnel: w270 -> [w280 w297 w306 w315 w348]
                  tunnel: w269 -> [w281 w298 w307 w316 w347]
                  tunnel: [w280 w296 w306 w315 w348] -> w268
                  tunnel: [w281 w295 w307 w316 w347] -> w267
                  tunnel: [w279 w291 w304 w313 w344] -> w266
                  tunnel: w265 -> [w279 w291 w304 w313 w343]
                  tunnel: [w278 Control2_MichaelVasmerDavidWise."Read R(T)" Control2_MichaelVasmerDavidWise."Read R(T)" Control2_MichaelVasmerDavidWise."Read R(T)" Control2_MichaelVasmerDavidWise."Read R(T)"] -> w264
                  tunnel: w263 -> [w277 w289 w302 w311 w326]
                  tunnel: [w276 w289 w302 w311 w326] -> w262
                  tunnel: [w274 w287 w301 w310 w321] -> w261
                  tunnel: [w273 w288 w300 w309 w320] -> w260
                  tunnel: w259 -> [w274 w287 w301 w310 w323]
                  tunnel: w258 -> [w273 w288 w300 w309 w322]
                  frame "Idle", Default {
                    n57 = global read "He3_Tlogger_Global 1.vi" "elapsed time (s)"() -> (w276:dbl)
                    n58 = Equal?(x=w277, y=w276) -> (x = y?=w275:bool)
                    n59 = case shown="True" w275 {
                      tunnel: [Control3_MichaelVasmerDavidWise."Read T" Control3_MichaelVasmerDavidWise."Idle"] -> w282
                      tunnel: [Control2_MichaelVasmerDavidWise."Read R(T)" Control2_MichaelVasmerDavidWise."Read R(T)"] -> w278
                      frame False {
                      }
                      frame True {
                      }
                    }
                  }
                  frame "Read Lockin" {
                    n60 = call-poly "Read.vi"("error in (no error)"=w297, "VISA resource name"=w298) -> ("error out"=w296:errorcluster, "Parameter Values"=w294:T4, "VISA resource name out"=w295:refnum<visa-resource-name>)  [unwired: 7 in]
                    n61 = Unbundle By Name(w294) -> ("X-Value"=w293:dbl, "Y-Value"=w292:dbl)
                    n62 = local write "V_output_Y_channel"(w292) -> ()
                    n63 = local write "V_output_X_channel"(w293) -> ()
                  }
                  frame "Read T" {
                    n64 = global read "He3_Tlogger_Global 1.vi" "Sample (sensor B) (K)"() -> (→"T 1":dbl)
                  }
                  frame "Read T 2" {
                    n65 = global read "He3_Tlogger_Global 1.vi" "Sample (sensor B) (K)"() -> (→"T 2":dbl)
                  }
                  frame "Write File" {
                    n66 = local read "T 1"() -> (w325:dbl)
                    n67 = local read "V_output_X_channel"() -> (w332:dbl)
                    n68 = local read "I_AC Amplitude (A)"() -> (w333:dbl)
                    n69 = Initialize Array(w325, 1 ("dimension size")) -> (w339:dbl[])
                    n70 = local read "T 2"() -> (w340:dbl)
                    n71 = Insert Into Array(array=w339, index=1, new element=w340) -> (w337:dbl[])
                    n72 = local read "V_output_Y_channel"() -> (w334:dbl)
                    n73 = Divide(x=w332, y=w333) -> (x/y=w324:dbl)
                    n74 = Insert Into Array(array=w337, index=2, new element=w324) -> (w336:dbl[])
                    n75 = Insert Into Array(array=w336, index=3, new element=w332) -> (w335:dbl[])
                    n76 = Build Array (concatenate)(w322, w324) -> (w320:dbl[])
                    n77 = Insert Into Array(array=w335, index=4, new element=w334) -> (w328:dbl[])
                    n78 = Build Array (concatenate)(w323, w325) -> (w321:dbl[])
                    n79 = Bundle(w321, w320) -> (→"R vs Temp":cluster{dbl[], dbl[]})  [unwired: 1 in]
                    n80 = call-poly <vilib>:"Write To Spreadsheet File.vi"("delimiter (\\t)"="," ("delimiter (\\t)"), "format (%.3f)"="%.11e", "append to file? (new file:F)"=TRUE, "1D data"=w328, "file path (dialog if empty)"=w343) -> ("new file path (Not A Path if cancelled)"=w344:path)  [unwired: 2 in, 1 out]
                  }
                }
              }
              event "Stop Sweep R(T)": Value Change {
                n81 = event-data() -> ()  [unwired: 1 in, 5 out]
                n82 = Get Date/Time In Seconds() -> (seconds since 1Jan1904=w354:timestamp)
                n83 = local read "File String Template 2"() -> (w355:string)
                n84 = Format Date/Time String(time format string (%c)="_PLOT_%H_%S", seconds (now)=w354) -> (date/time string=w356:string)  [unwired: 1 in]
                n85 = Concatenate Strings(w355, w356) -> (w358:string)
                n86 = String To Path(string=w358) -> (path=w351:path)
                n87 = invoke on="R vs Temp" class="XYGraph (strict)" method="Export Image"("FileType"=enum32{"BMP", "EPS", "EMF", "PICT"}."BMP" ("File Type"), "Target"=enum32{"File", "Clipboard"}."File", "Path"=w351) -> ()  [unwired: 5 in, 8 out]
              }
              event "Force Measurement": Value Change {
                n88 = event-data() -> ()  [unwired: 1 in, 6 out]
              }
            }
          }
          frame "Shutdown All" {
            n89 = local read "Keithley on (default false)"() -> (w376:bool)
            n90 = local read "Lock In On (default false)"() -> (w371:bool)
            n91 = case shown="False" w376 {
              tunnel: w375 -> [_ w385]
              tunnel: w374 -> [w382 w384]
              tunnel: [w382 w383] -> w370
              frame False {
              }
              frame True {
                w388 = FALSE  # Enable Output
                n92 = call "Enable Output.vi"("error in (no error)"=w385, "Enable Output (T: Enable)"=w388, "VISA resource name"=w384) -> ("error out"=w387:errorcluster, "VISA resource name out"=w383:refnum<visa-resource-name>)  [unwired: 7 in]
                n93 = local write "Keithley on (default false)"(FALSE ("Keithley on")) -> ()
                n94 = call "Close.vi"("error in (no error)"=w387, "VISA resource name"=w383) -> ()  [unwired: 9 in, 1 out]
              }
            }
            n95 = case shown="True" w371 {
              tunnel: w373 -> [w378 w379]
              tunnel: w372 -> [_ w381]
              tunnel: [w378 w379] -> w369
              frame False {
              }
              frame True {
                n96 = call "Close.vi"("error in (no error)"=w381, "VISA resource name"=w379) -> ()  [unwired: 9 in, 1 out]
                n97 = local write "Lock In On (default false)"(FALSE ("Lock In On (default false)")) -> ()
              }
            }
          }
          frame "Shutdown Lock in" {
            n98 = call "Close.vi"("error in (no error)"=w394, "VISA resource name"=w390) -> ()  [unwired: 9 in, 1 out]
            n99 = local write "Lock In On (default false)"(FALSE ("Lock In On (default false)")) -> ()
          }
          frame "Open File" {
            w435 = TRUE  # append to file?
            w433 = ","  # delimiter (\t)
            # "Write Header"
            # "Write Channel Names"
            n100 = Get Date/Time In Seconds() -> (seconds since 1Jan1904=w400:timestamp)
            n101 = Format Date/Time String(time format string (%c)="%H_%M_%S", seconds (now)=w400) -> (date/time string=w399:string)  [unwired: 1 in]
            n102 = Concatenate Strings("File String Template", w399) -> (w429:string)
            n103 = Initialize Array("R_series", 1 ("dimension size")) -> (w426:string[])
            n104 = Concatenate Strings(w429, ".csv" ("string")) -> (w430:string)
            n105 = Insert Into Array(array=w426, index=1, new element="100") -> (w425:string[])
            n106 = String To Path(string=w430) -> (path=w432:path)
            n107 = Insert Into Array(array=w425, index=2, new element="kiloOhms") -> (w418:string[])
            n108 = Initialize Array("B(T)", 1 ("dimension size")) -> (w417:string[])
            n109 = Insert Into Array(array=w417, index=1, new element="R(Ohms)") -> (w416:string[])
            n110 = call-poly <vilib>:"Write To Spreadsheet File.vi"("delimiter (\\t)"="," ("delimiter (\\t)"), "append to file? (new file:F)"=FALSE, "1D data"=w418, "file path (dialog if empty)"=w432) -> ("new file path (Not A Path if cancelled)"=w434:path)  [unwired: 3 in, 1 out]
            n111 = Insert Into Array(array=w416, index=2, new element="T(K)") -> (w403:string[])
            n112 = Insert Into Array(array=w403, index=3, new element="V (X)") -> (w402:string[])
            n113 = Insert Into Array(array=w402, index=4, new element="V (Y)") -> (w401:string[])
            n114 = call-poly <vilib>:"Write To Spreadsheet File.vi"("delimiter (\\t)"=w433, "append to file? (new file:F)"=w435, "1D data"=w401, "file path (dialog if empty)"=w434) -> ("new file path (Not A Path if cancelled)"=w409:path)  [unwired: 3 in, 1 out]
          }
          frame "Write File" {
            n115 = local read "Magnetic Field (T)"() -> (w442:dbl)
            n116 = local read "V_output_Y_channel"() -> (w447:dbl)
            n117 = local read "V_output_X_channel"() -> (w448:dbl)
            n118 = local read "Temperature (K)"() -> (w450:dbl)
            n119 = local read "I_AC Amplitude (A)"() -> (w449:dbl)
            n120 = Initialize Array(w442, 1 ("dimension size")) -> (w460:dbl[])
            n121 = Divide(x=w448, y=w449) -> (x/y=w441:dbl)
            n122 = Insert Into Array(array=w460, index=1, new element=w441) -> (w459:dbl[])
            n123 = Insert Into Array(array=w459, index=2, new element=w450) -> (w453:dbl[])
            n124 = Insert Into Array(array=w453, index=3, new element=w448) -> (w452:dbl[])
            n125 = Insert Into Array(array=w452, index=4, new element=w447) -> (w451:dbl[])
            n126 = Build Array (concatenate)(w444, w442) -> (w440:dbl[])
            n127 = Build Array (concatenate)(w443, w441) -> (w439:dbl[])
            n128 = Bundle(w440, w439) -> (→"R vs B":cluster{dbl[], dbl[]})  [unwired: 1 in]
            n129 = call-poly <vilib>:"Write To Spreadsheet File.vi"("delimiter (\\t)"="," ("delimiter (\\t)"), "format (%.3f)"="%.16e", "append to file? (new file:F)"=TRUE, "1D data"=w451, "file path (dialog if empty)"=w461) -> ("new file path (Not A Path if cancelled)"=w446:path)  [unwired: 2 in, 1 out]
            "Array" <- w444
          }
          frame "Open File 2" {
            w511 = TRUE  # append to file?
            w509 = ","  # delimiter (\t)
            # "Write Header"
            # "Write Channel Names"
            n130 = Get Date/Time In Seconds() -> (seconds since 1Jan1904=w478:timestamp)
            n131 = Format Date/Time String(time format string (%c)="%H_%M_%S", seconds (now)=w478) -> (date/time string=w477:string)  [unwired: 1 in]
            n132 = Concatenate Strings("File String Template 2", w477) -> (w506:string)
            n133 = Initialize Array("R_series", 1 ("dimension size")) -> (w503:string[])
            n134 = Concatenate Strings(w506, ".csv" ("string")) -> (w507:string)
            n135 = Insert Into Array(array=w503, index=1, new element="100") -> (w502:string[])
            n136 = String To Path(string=w507) -> (path=w508:path)
            n137 = Insert Into Array(array=w502, index=2, new element="kiloOhms") -> (w495:string[])
            n138 = Initialize Array("T_1(K)", 1 ("dimension size")) -> (w494:string[])
            n139 = Insert Into Array(array=w494, index=1, new element="T_2(K)") -> (w493:string[])
            n140 = call-poly <vilib>:"Write To Spreadsheet File.vi"("delimiter (\\t)"="," ("delimiter (\\t)"), "append to file? (new file:F)"=FALSE, "1D data"=w495, "file path (dialog if empty)"=w508) -> ("new file path (Not A Path if cancelled)"=w510:path)  [unwired: 3 in, 1 out]
            n141 = Insert Into Array(array=w493, index=2, new element="R(Ohms)") -> (w482:string[])
            n142 = Insert Into Array(array=w482, index=3, new element="V (X)") -> (w481:string[])
            n143 = Insert Into Array(array=w481, index=4, new element="V (Y)") -> (w480:string[])
            n144 = call-poly <vilib>:"Write To Spreadsheet File.vi"("delimiter (\\t)"=w509, "append to file? (new file:F)"=w511, "1D data"=w480, "file path (dialog if empty)"=w510) -> ("new file path (Not A Path if cancelled)"=w472:path)  [unwired: 3 in, 1 out]
          }
        }
      }
      event "Shutdown": Value Change {
        n145 = event-data() -> ()  [unwired: 1 in, 6 out]
      }
      event "Sweep R(T)": Value Change {
        n146 = event-data() -> ()  [unwired: 1 in, 6 out]
        n147 = local write "True  = R(B)\nFalse = R(T)"(FALSE ("True  = R(B)\nFalse = R(T)")) -> ()
      }
      event "Sweep R(B)": Value Change {
        n148 = event-data() -> ()  [unwired: 1 in, 6 out]
        n149 = local write "True  = R(B)\nFalse = R(T)"(TRUE ("True  = R(B)\nFalse = R(T)")) -> ()
      }
    }
    "Inner State Machine" <- w27
    "Outer State Machine" <- w41
  }
